vi "Update Cluster Controls.vi"(8 "Cluster Indicator Indexes":i32[](array[numeric]), 9 "Indicators In":refnum<class "Object.lvclass">[](array[class]), 10 "Cluster Control Indexes":i32[](array[numeric]), 11 "Controls In":refnum<class "Object.lvclass">[](array[class])) -> (2 "Indicators Out":refnum<class "Object.lvclass">[](array[class]), 3 "Controls Out":refnum<class "Object.lvclass">[](array[class]))   [LabVIEW 2017, in "Front Panel Publisher.lvlib" / "Web Front Panel.lvclass"]
uses:
  Web Front Panel.lvclass
  Front Panel Objects/Cluster_class/Front Panel Objects/String_class/Cluster.lvclass
  Front Panel Objects/Object_class/Object.lvclass
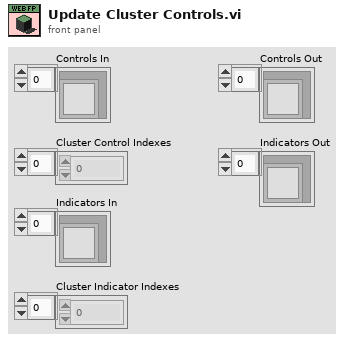
[diagram p1: front panel]
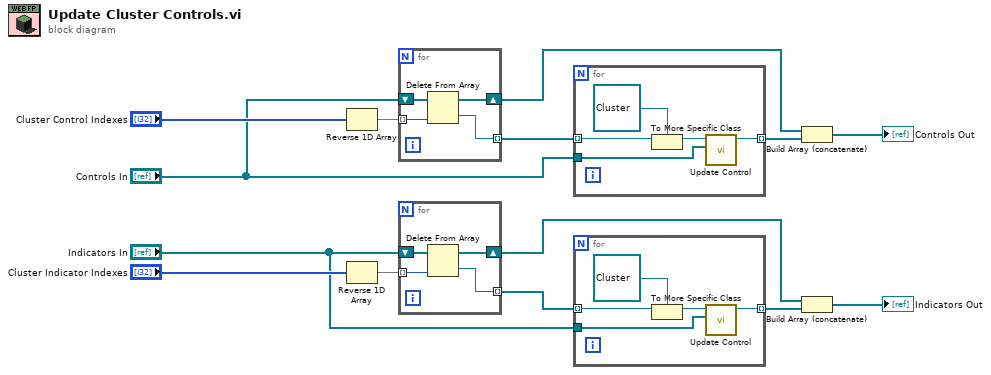
[diagram p0: block diagram]
diagram:
  n1 = Reverse 1D Array(array="Cluster Control Indexes") -> (reversed array=w5:i32[])
  n2 = Reverse 1D Array(array="Cluster Indicator Indexes") -> (reversed array=w10:i32[])
  n3 = for "For Each element to delete" {
    tunnel: w5 -> [w18] mode=indexing
    shift-right: [w17] -> w3
    shift-left: "Controls In" -> [w16]
    tunnel: [w15] -> w2 mode=indexing
    n4 = Delete From Array(array=w16, index=w18) -> (deleted portion=w15:refnum<class "Object.lvclass">, array with subset deleted=w17:refnum<class "Object.lvclass">[])  [unwired: 1 in]
  }
  n5 = for "For Each element to delete" {
    tunnel: w10 -> [w22] mode=indexing
    shift-right: [w21] -> w7
    shift-left: "Indicators In" -> [w20]
    tunnel: [w19] -> w6 mode=indexing
    n6 = Delete From Array(array=w20, index=w22) -> (deleted portion=w19:refnum<class "Object.lvclass">, array with subset deleted=w21:refnum<class "Object.lvclass">[])  [unwired: 1 in]
  }
  n7 = for {
    tunnel: [w25] -> w14 mode=indexing
    tunnel: w2 -> [w24] mode=indexing
    tunnel: "Controls In" -> [w23]
    n8 = To More Specific Class(target class=refnum<class "Cluster.lvclass"> refnum ("Control out"), reference=w24) -> (specific class reference=w27:refnum<class "Cluster.lvclass">)  [unwired: 1 in, 1 out]
    n9 = call "Update Control.vi"("Updated Controls"=w23, "Cluster in"=w27) -> ("Cluster out"=w25:refnum<class "Cluster.lvclass">)  [unwired: 8 in, 1 out]
  }
  n10 = for {
    tunnel: [w30] -> w12 mode=indexing
    tunnel: w6 -> [w29] mode=indexing
    tunnel: "Indicators In" -> [w28]
    n11 = To More Specific Class(target class=refnum<class "Cluster.lvclass"> refnum ("Control out"), reference=w29) -> (specific class reference=w32:refnum<class "Cluster.lvclass">)  [unwired: 1 in, 1 out]
    n12 = call "Update Control.vi"("Updated Controls"=w28, "Cluster in"=w32) -> ("Cluster out"=w30:refnum<class "Cluster.lvclass">)  [unwired: 8 in, 1 out]
  }
  n13 = Build Array (concatenate)(w3, w14) -> (→"Controls Out":refnum<class "Object.lvclass">[])
  n14 = Build Array (concatenate)(w7, w12) -> (→"Indicators Out":refnum<class "Object.lvclass">[])
